vi "CR-字符检测处理函数as.vi"(0 "Image in":T6(plugin-control), 1 "字符识别参数":T5={"Parameters (OCR/OCV 1)"={"Threshold Data"={"Method"=enum."Local", "Looking for"=1, "Color Mode"=0, "Kernel Size"={"Width"=32, "Height"=32}, "Ranges"=[{"Min"=1, "Max"=255}]}, "Reject Border"=TRUE, "Number Of Erosions"=0, "Size & Spacing"={"Segment Algorithm"=0, "Min Bounding Rect Width"=1, "Max Bounding Rect Width"=65536, "Min Bounding Rect Height"=1, "Max Bounding Rect Height"=65536, "Min Character Size"=20, "Max Character Size"=65536, "Min Char Spacing"=1, "Max Horiz Element Spacing"=1, "Max Vert Element Spacing"=0, "Max Space Distance"=65536}, "Read Options"={"Read Strategy"=1, "Read Resolution"=2, "Scale Dependant"=FALSE, "Aspect Ratio"=400, "Acceptance Level"=700, "Substitution Character"="?", "MultiLine"=TRUE}, "Valid Characters"=[], "Use Text Pattern"=FALSE, "Orientation"=0, "# Lines Expected"=0, "Number of Blocks"=4}, "Rectangle"={"Left"=0, "Top"=0, "Right"=0, "Bottom"=0, "Rotation"=0.0}, "字符长度判定"=0.0, "Reference System"={"Origin"={"X"=1245.2058, "Y"=1038.7815}, "Angle (deg)"=0.021420227, "Axis Reference"=0}, "File Path (字符库)"=path "D:/Inspect System/Source Code/Template Program/字符模板.abc", "File Path (连接件模板)"=path "D:/Inspect System/Source Code/Template Program/字符检测定位模板.png", "Url"="http://10.6.1.31:8080/MesInnerpackLineIO.asmx", "accessKey"="a45b2d3334ffs_\na45b2d3334ffs_"} {"Reference System"."Axis Reference" items=["Direct", "Indirect"]; "Rectangle"."Rotation" min=-90.0 max=90.0 step=1.0 format="%.2f"; "Rectangle"."Left" scale=0.0..1024.0; "Rectangle"."Right" scale=0.0..1024.0; "Parameters (OCR/OCV 1)"."Threshold Data"."Looking for" items=["Light on Dark", "Dark on Light"]; "Parameters (OCR/OCV 1)"."Threshold Data"."Color Mode" items=["RGB", "HSL", "HSV", "HSI"]; "Parameters (OCR/OCV 1)"."Size & Spacing"."Segment Algorithm" items=["None", "Shortest Segment", "Legacy Auto Split"]; "Parameters (OCR/OCV 1)"."Read Options"."Read Strategy" items=["Aggressive", "Conservative"]; "Parameters (OCR/OCV 1)"."Read Options"."Read Resolution" items=["Low", "Medium", "High"]; "Parameters (OCR/OCV 1)"."Valid Characters"."Pre-defined characters" items=["Any Character", "User-defined Characters", "Alphabetic", "Alphanumeric", "Uppercase Letters", "Lowercase Letters", "Decimal Digits", "Hexadecimal Digits", "Pattern", "Force Space"]; "Parameters (OCR/OCV 1)"."Orientation" items=["Baseline inside", "Baseline outside"]}, 5 "error in (no error)":errorcluster caption="错误输入（无错误）", 7 "CCD1字符定位参数":T4={"Rectangle"={"Left"=9, "Top"=176, "Right"=891, "Bottom"=836, "Rotation"=0.0}, "Settings"={"Curve Parameters"={"Extraction Mode"=0, "Edge Threshold"=35, "Edge Filter Size"=1, "Min Length"=25, "Row Search Step Size"=15, "Col Search Step Size"=15, "Max Endpoint Gap"=10, "Closed"=FALSE, "Subpixel"=FALSE}, "Match Mode"={"Rotation"=TRUE, "Scale"=FALSE, "Occlusion"=TRUE, "Reserved 1"=FALSE, "Reserved 2"=FALSE, "Reserved 3"=FALSE}, "Range Settings"=[{"Match Constraints"=0, "Min"=-17.0, "Max"=17.0}], "Number of Matches"=1, "Minimum Match Score"=400.0, "SubPixel Accuracy"=FALSE, "Adv. Geometric Match Options 2"=[{"Setup Data Item"=21, "Item Value"=0.0}]}, "Template File Path"=path "D:/Inspect System/Source Code/SubVIs/字符检测VI/aaaa.png"} {"Settings"."Curve Parameters"."Extraction Mode" items=["Normal", "Uniform Regions"]; "Settings"."Curve Parameters"."Edge Filter Size" items=["Fine", "Normal", "Contour Tracing"]; "Settings"."Curve Parameters"."Max Endpoint Gap" min=0; "Settings"."Curve Parameters"."Col Search Step Size" min=1 max=255 step=1; "Settings"."Curve Parameters"."Row Search Step Size" min=1 max=255 step=1; "Settings"."Curve Parameters"."Min Length" min=0; "Settings"."Curve Parameters"."Edge Threshold" min=1 max=350 step=1; "Settings"."Range Settings"."Max" format="%.2f"; "Settings"."Range Settings"."Min" format="%.2f"; "Settings"."Range Settings"."Match Constraints" items=["Rotation Angle (degrees)", "Scale Factor (%)", "Occlusion (%)"]; "Settings"."Adv. Geometric Match Options 2"."Setup Data Item" items=["Curve Extraction Mode", "Curve Edge Threshold", "Curve Edge Filter Size", "Min Curve Length", "Curve Row Search Step Size", "Curve Col Search Step Size", "Curve Max Endpoint Gap", "Extract Closed Curves", "Enable Subpixel Curve Extraction", "Enable Correlation Score", "Enable Subpixel Accuracy", "Subpixel Iterations", "Subpixel Tolerance", "Initial Match List Length", "Enable Target Template Curve Score", "Min Match Separation Distance", "Min Match Separation Angle", "Min Match Separation Scale", "Max Match Overlap", "Enable Coarse Result", "Enable Calibration Support", "Enable Contrast Reversal", "Search Strategy", "Refinement Match Factor", "Subpixel Match Factor"]; "Rectangle"."Rotation" format="%.2f"; "Rectangle"."Left" scale=0.0..1024.0; "Rectangle"."Right" scale=0.0..1024.0}) -> (12 "模板匹配OK/NG":bool, 14 "Image out":T6(plugin-control), 16 "Data":string, 17 "字符方向判定结果":bool, 18 "结果":bool, 19 "error out":errorcluster caption="错误输出")   [LabVIEW 2017]
uses:
  <vilib>/vision/Pattern Matching.llb/IMAQ Curve Parameters.ctl
  <vilib>/vision/Pattern Matching.llb/IMAQ Match Range Setting.ctl
  <vilib>/vision/NI_Vision_Development_Module.lvlib
panel:
  in  "Bounding Box 3":cluster{"x":sgl, "y":sgl}[](array[cluster])
  out "Bounding Box 2":cluster{"x":sgl, "y":sgl}[](array[cluster])
  out "Bounding Box":cluster{"x":sgl, "y":sgl}[](array[cluster])
  # "D:\\Inspect System -2\\Source Code\\Template Program\\程序1\\字符模板.abc"
  # "Range"
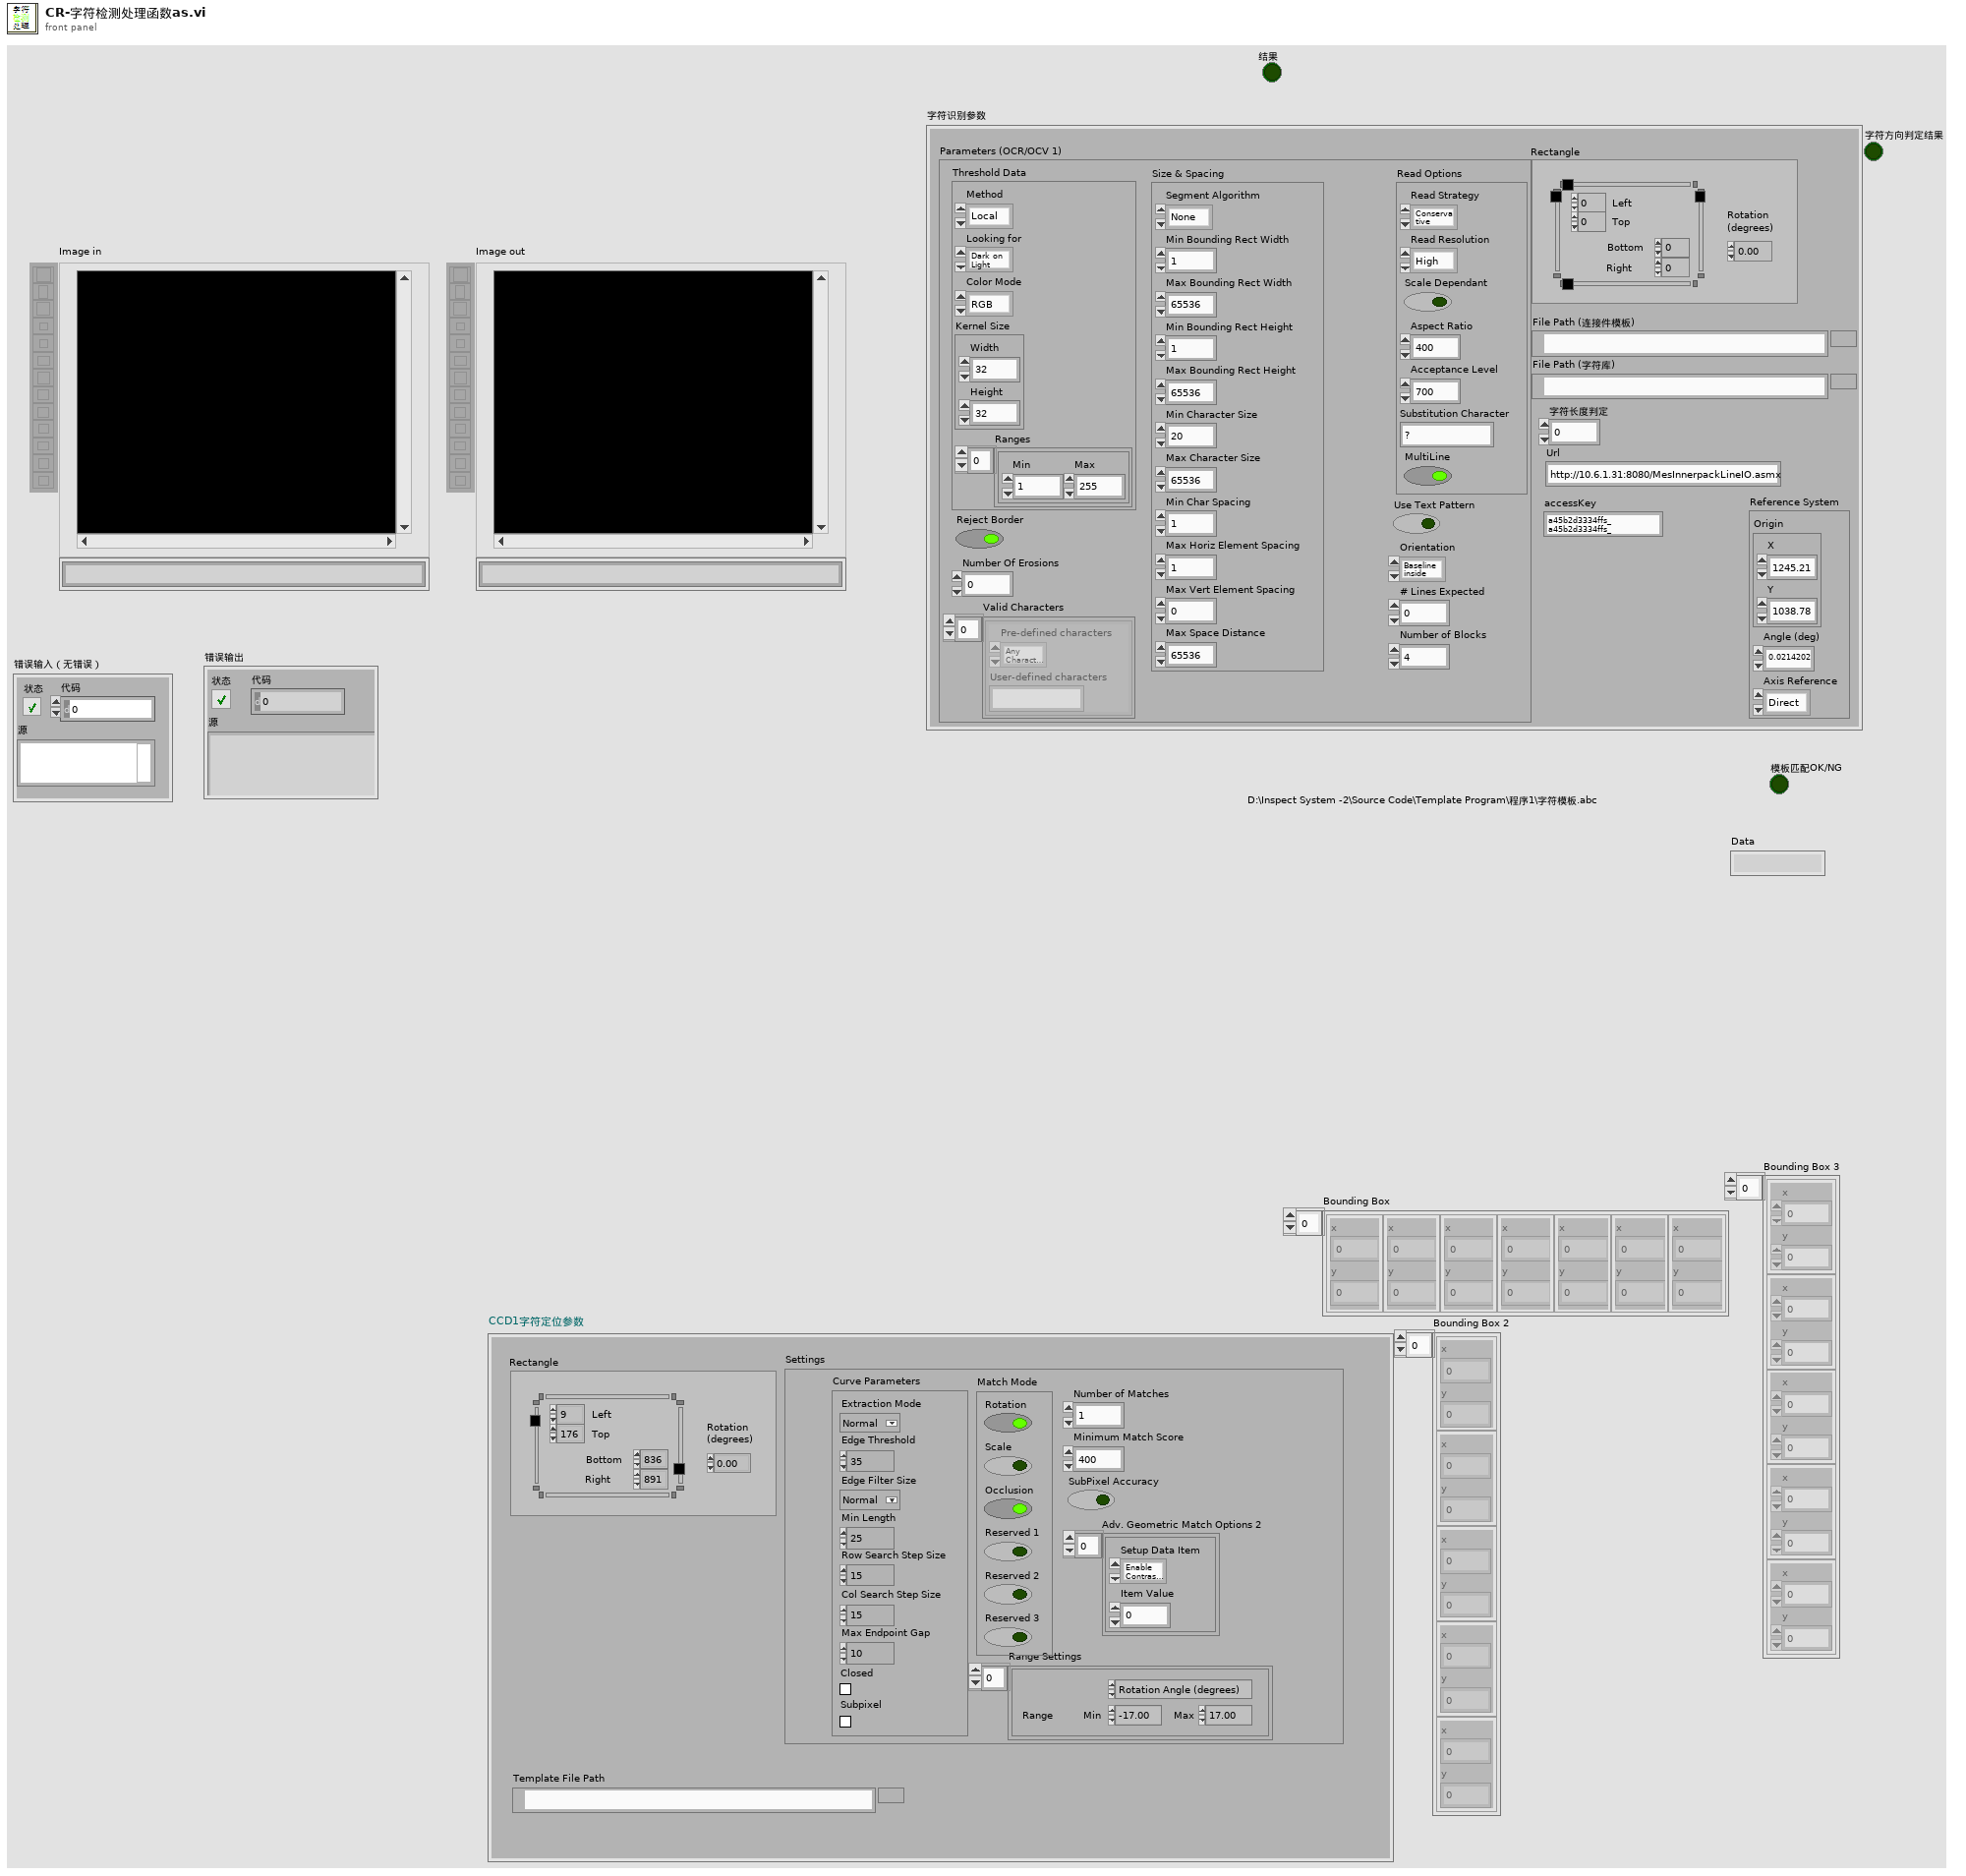
[diagram p1: front panel]
types:
  T1 = typedef "IMAQ Rectangle" = cluster{"Left":i32, "Top":i32, "Right":i32, "Bottom":i32, "Rotation":dbl}
  T2 = typedef "IMAQ Curve Parameters.ctl" = cluster{"Extraction Mode":u32, "Edge Threshold":i32, "Edge Filter Size":u32, "Min Length":i32, "Row Search Step Size":i32, "Col Search Step Size":i32, "Max Endpoint Gap":i32, "Closed":bool, "Subpixel":bool}
  T3 = typedef "IMAQ Match Range Setting.ctl" = cluster{"Match Constraints":u32, "Min":dbl, "Max":dbl}
  T4 = cluster{"Rectangle":T1, "Settings":cluster{"Curve Parameters":T2, "Match Mode":cluster{"Rotation":bool, "Scale":bool, "Occlusion":bool, "Reserved 1":bool, "Reserved 2":bool, "Reserved 3":bool}, "Range Settings":T3[], "Number of Matches":i32, "Minimum Match Score":sgl, "SubPixel Accuracy":bool, "Adv. Geometric Match Options 2":cluster{"Setup Data Item":u16, "Item Value":dbl}[]}, "Template File Path":path}
  T5 = cluster{"Parameters (OCR/OCV 1)":cluster{"Threshold Data":cluster{"Method":enum16{"Fixed Range", "Uniform", "Linear", "Non Linear", "Local", "Color"}, "Looking for":u32, "Color Mode":u32, "Kernel Size":cluster{"Width":i32, "Height":i32}, "Ranges":cluster{"Min":i32, "Max":i32}[]}, "Reject Border":bool, "Number Of Erosions":i32, "Size & Spacing":cluster{"Segment Algorithm":u16, "Min Bounding Rect Width":i32, "Max Bounding Rect Width":i32, "Min Bounding Rect Height":i32, "Max Bounding Rect Height":i32, "Min Character Size":i32, "Max Character Size":i32, "Min Char Spacing":i32, "Max Horiz Element Spacing":i32, "Max Vert Element Spacing":i32, "Max Space Distance":i32}, "Read Options":cluster{"Read Strategy":i32, "Read Resolution":i32, "Scale Dependant":bool, "Aspect Ratio":i32, "Acceptance Level":i32, "Substitution Character":string, "MultiLine":bool}, "Valid Characters":cluster{"Pre-defined characters":i32, "User-defined characters":string}[], "Use Text Pattern":bool, "Orientation":u32, "# Lines Expected":u32, "Number of Blocks":i32}, "Rectangle":T1, "字符长度判定":dbl, "Reference System":cluster{"Origin":cluster{"X":sgl, "Y":sgl}, "Angle (deg)":sgl, "Axis Reference":u32}, "File Path (字符库)":path, "File Path (连接件模板)":path, "Url":string, "accessKey":string}
  T6 = typedef "IMAQ Image.ctl" = refnum<image>
  T7 = cluster{"Rotation Mode":enum32{"Unlimited", "0 Degrees", "90 Degrees", "180 Degrees", "270 Degrees"}, "Skip Location?":bool, "Edge Threshold":u32, "Demodulation Mode":i32, "Cell Sample Size":i32, "Cell Filter Mode":i32, "Skew Degrees Allowed":u32}
  T8 = cluster{"Left":i32, "Top":i32, "Right":i32, "Bottom":i32}
  T9 = cluster{"Global Rectangle":i32[], "Contours":cluster{"ID":enum32{"External", "Internal"}, "Type":u32, "Coordinates":i32[]}[]}
  T10 = cluster{"Desired Font (Application)":enum16{"User-specified Font", "Application Font", "System Font", "Dialog Font"}, "[User-specified Font]":cluster{"Font Name":string, "Size":i16, "Strikeout?":bool, "Italic?":bool, "Underline?":bool, "Outline?":bool, "Shadow?":bool, "Bold?":bool, "Rotation Angle":dbl}, "Horizontal Alignment":i16, "Vertical Alignment":i16}
  T11 = typedef "ROI Descriptor" = cluster{"Global Rectangle":i32[], "Contours":cluster{"ID":enum32{"External", "Internal"}, "Type":u32, "Coordinates":i32[]}[]}
  T12 = typedef "IMAQ GM Match Report.ctl" = cluster{"Position":cluster{"x":sgl, "y":sgl}, "Angle":sgl, "Scale":sgl, "Score":sgl, "Bounding Box":cluster{"x":sgl, "y":sgl}[], "Contrast Reversed":bool, "Occlusion %":sgl, "Template Target Curve Score":sgl, "Target Template Curve Score":sgl, "Correlation Score":sgl}
  T13 = cluster{"Reference System":cluster{"Origin":cluster{"X":sgl, "Y":sgl}, "Angle (deg)":sgl, "Axis Reference":u32}, "Measurement System":cluster{"Origin":cluster{"X":sgl, "Y":sgl}, "Angle (deg)":sgl, "Axis Reference":u32}}
  T14 = cluster{"Position":cluster{"x":sgl, "y":sgl}, "Angle":sgl, "Scale":sgl, "Score":sgl, "Bounding Box":cluster{"x":sgl, "y":sgl}[]}[]
  T15 = cluster{"Position":cluster{"x":sgl, "y":sgl}, "Angle":sgl, "Scale":sgl, "Score":sgl, "Bounding Box":cluster{"x":sgl, "y":sgl}[]}
  T16 = cluster{"Origin":cluster{"X":sgl, "Y":sgl}, "Angle (deg)":sgl, "Axis Reference":u32}
  T17 = typedef "QR Code Report.ctl" = cluster{"Found?":bool, "Data":string, "Bounding Box":cluster{"x":sgl, "y":sgl}[], "Errors Corrected":u32, "Dimensions (Rows/Cols)":u32, "Version":u32, "QR Model":T18, "Stream Mode":T19, "Barcode Polarity":T20, "Mirrored?":bool, "Append Stream Position":u32, "Size of Append Stream":u32, "First EAN-128 ID":i32, "First Alternate Language ID":i32, "Append Stream ID":u32, "Minimum Edge Strength":u32, "Demodulation Mode":T21, "Cell Sample Size":T22, "Cell Filter Mode":T23}
  T18 = typedef "QR Code Model Type.ctl" = i32
  T19 = typedef "QR Code Stream Mode Type.ctl" = i32
  T20 = typedef "Data Matrix Polarity.ctl" = i32
  T21 = typedef "Demodulation Mode.ctl" = i32
  T22 = typedef "Cell Sample Size.ctl" = i32
  T23 = typedef "Cell Filter Mode.ctl" = i32
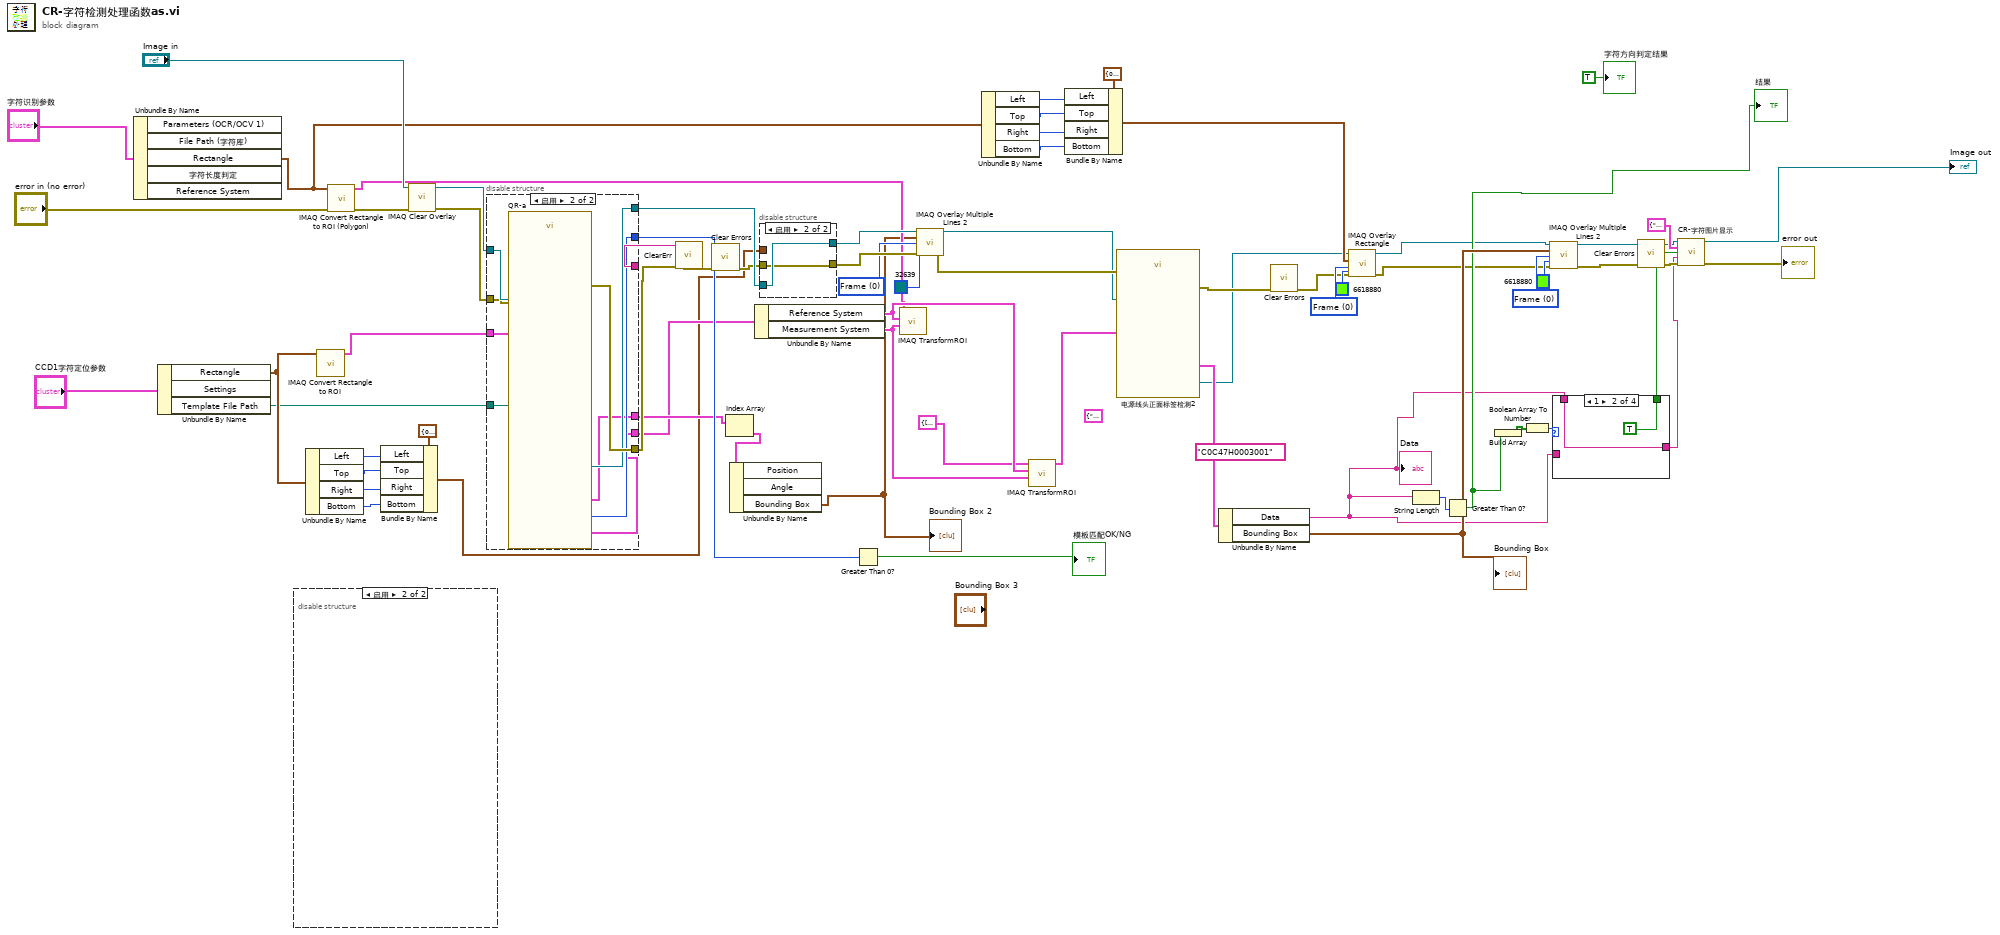
[diagram p0: block diagram]
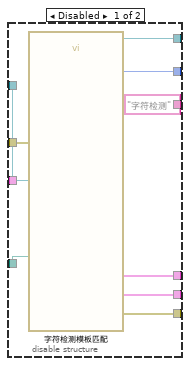
[diagram p2: hidden frame]
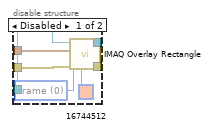
[diagram p3: hidden frame]
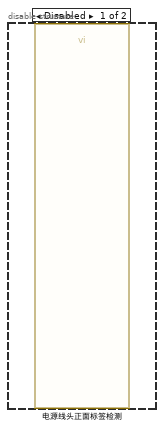
[diagram p4: hidden frame]
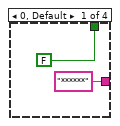
[diagram p5: hidden frame]
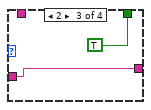
[diagram p6: hidden frame]
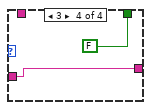
[diagram p7: hidden frame]
diagram:
  (unwired) T7 {"Rotation Mode"=enum."Unlimited", "Skip Location?"=FALSE, "Edge Threshold"=11, "Demodulation Mode"=1, "Cell Sample Size"=3, "Cell Filter Mode"=2, "Skew Degrees Allowed"=5} ("QR Search Options (2D Barcode Reader 1)")
  w20 = u32 0 items=["Frame", "Fill"] ("Drawing Mode (Frame)")
  w22 = u32 0 items=["Frame", "Fill"] ("Drawing Mode (Frame)")
  (unwired) "C0C47H0003001" ("Data")
  w57 = u32 0 items=["Frame", "Fill"] ("Drawing Mode (Frame)")
  n1 = Unbundle By Name("字符识别参数") -> ("Rectangle"=w5:T1)  [unwired: 4 out]
  n2 = Unbundle By Name("CCD1字符定位参数") -> ("Rectangle"=w41:T1, "Template File Path"=w33:path)  [unwired: 1 out]
  n3 = disable-structure shown="启用" {
    frame Disabled {
      n4 = call "电源线头正面标签检测"() -> ()  [unwired: 21 in, 7 out]
    }
    frame Enabled {
    }
  }
  n5 = Unbundle By Name(w41) -> ("Left"=w40:i32, "Top"=w39:i32, "Right"=w38:i32, "Bottom"=w37:i32)
  n6 = call "IMAQ Convert Rectangle to ROI"("Rectangle"=w41) -> ("ROI Descriptor"=w15:T11)  [unwired: 8 in, 1 out]
  n7 = call "IMAQ Convert Rectangle to ROI (Polygon)"("error in (no error)"="error in (no error)", "Rectangle"=w5) -> ("error out"=w45:errorcluster, "ROI Descriptor"=w13:T11)  [unwired: 6 in, 1 out]
  n8 = Bundle By Name(cluster=T8 {"Left"=0, "Top"=0, "Right"=0, "Bottom"=0} ("Rectangle"), "Left"=w40, "Top"=w39, "Right"=w38, "Bottom"=w37) -> (w11:T8)
  n9 = call "IMAQ Clear Overlay"("error in (no error)"=w45, "Image"="Image in") -> ("error out"=w34:errorcluster, "Image Out"=w28:T6)  [unwired: 8 in]
  n10 = disable-structure shown="启用" {
    disable-tunnel: [w79 w83] -> w63
    disable-tunnel: ["字符检测" ("运行位置") _] -> w36
    disable-tunnel: w34 -> [w77 w86]
    disable-tunnel: w33 -> [w76 w88]
    disable-tunnel: [w75 w85] -> w32
    disable-tunnel: [w74 w81] -> w31
    disable-tunnel: [w73 w82] -> w30
    disable-tunnel: [w72 w84] -> w29
    disable-tunnel: w28 -> [w71 w87]
    disable-tunnel: w15 -> [_ w80]
    frame Disabled {
      n11 = call "字符检测模板匹配.vi"("Image In"=w71, "Template File Path (Geometric Matching 1)"=w76, "error in"=w77) -> ("Image Out"=w72:T6, "Calibrated Matches (Geometric Matching 1)"=w74:T12[], "Number of Matches (Geometric Matching 1)"=w79:i32, "Coordinate System Out (Set Coordinate System 1)"=w73:T13, "error out"=w75:errorcluster)  [unwired: 19 in, 1 out]
    }
    frame Enabled {
      n12 = call "QR-a.vi"("Image In"=w87, "Template File Path (Pattern Matching 1)"=w88, "error in"=w86, "ROI Descriptor (2D Barcode Reader 1)"=w80) -> ("Image Out"=w84:T6, "Calibrated Matches (Pattern Matching 1)"=w81:T14, "Number of Matches (Pattern Matching 1)"=w83:i32, "Coordinate System Out (Set Coordinate System 1)"=w82:T13, "error out"=w85:errorcluster)  [unwired: 16 in, 3 out]
    }
  }
  n13 = call "ClearErr.vi"("error in (no error)"=w32, "运行位置"=w36) -> ("error out"=w35:errorcluster)  [unwired: 9 in]
  n14 = call <vilib>:"Clear Errors.vi"("error in (no error)"=w35) -> ("error out"=w24:errorcluster)  [unwired: 5 in, 1 out]
  n15 = Index Array(array=w31) -> (element=w44:T15)  [unwired: 1 in]
  n16 = Unbundle By Name(w44) -> ("Bounding Box"=w1:cluster{"x":sgl, "y":sgl}[])  [unwired: 2 out]
  "Bounding Box 2" <- w1
  n17 = Unbundle By Name(w30) -> ("Reference System"=w26:T16, "Measurement System"=w27:T16)
  n18 = disable-structure shown="启用" {
    disable-tunnel: w11 -> [w95 _]
    disable-tunnel: w29 -> [w94 w97]
    disable-tunnel: [w93 w97] -> w25
    disable-tunnel: w24 -> [w92 w96]
    disable-tunnel: [w89 w96] -> w23
    frame Disabled {
      w91 = u32 0 items=["Frame", "Fill", "Highlight"] ("Drawing Mode (Frame)")
      n19 = call "IMAQ Overlay Rectangle"("Color"=u32 16744512, "error in (no error)"=w92, "Drawing Mode (Frame)"=w91, "Rectangle"=w95, "Image"=w94) -> ("error out"=w89:errorcluster, "Image Out"=w93:T6)  [unwired: 5 in]
    }
    frame Enabled {
    }
  }
  n20 = Greater Than 0?(x=w63) -> (x > 0?=→"模板匹配OK/NG":bool)
  n21 = call "IMAQ TransformROI"("New Reference"=w27, "Base Reference"=w26, "ROI Descriptor"=w13) -> ()  [unwired: 7 in, 2 out]
  n22 = call "IMAQ Overlay Multiple Lines 2"("Image"=w25, "Line End Points"=w1, "Drawing Mode (Frame)"=w22, "Color"=u32 32639, "error in (no error)"=w23) -> ("Image Out"=w62:T6, "error out"=w66:errorcluster)  [unwired: 9 in]
  n23 = Unbundle By Name(w5) -> ("Left"=w9:i32, "Top"=w8:i32, "Right"=w7:i32, "Bottom"=w6:i32)
  n24 = call "IMAQ TransformROI"("New Reference"=w27, "Base Reference"=w26, "ROI Descriptor"=T9 {"Global Rectangle"=[579, 508, 906, 745], "Contours"=[{"ID"=enum."External", "Type"=3, "Coordinates"=[579, 508, 906, 745]}]} ("ROI Descriptor (2D Barcode Reader 1)")) -> ("ROI Descriptor out"=w14:T11)  [unwired: 7 in, 1 out]
  n25 = Bundle By Name(cluster=T8 {"Left"=0, "Top"=0, "Right"=0, "Bottom"=0} ("Rectangle"), "Left"=w9, "Top"=w8, "Right"=w7, "Bottom"=w6) -> (w4:T8)
  n26 = call "电源线头正面标签检测2"("Image In"=w62, "error in"=w66, "ROI Descriptor (2D Barcode Reader 1)"=w14) -> ("Image Out"=w3:T6, "QR Barcode Report (2D Barcode Reader 1)"=w61:T17, "error out"=w50:errorcluster)  [unwired: 22 in]
  n27 = Unbundle By Name(w61) -> ("Data"=w2:string, "Bounding Box"=w56:cluster{"x":sgl, "y":sgl}[])
  "Data" <- w2
  "Bounding Box" <- w56
  n28 = call <vilib>:"Clear Errors.vi"("error in (no error)"=w50) -> ("error out"=w18:errorcluster)  [unwired: 5 in, 1 out]
  n29 = call "IMAQ Overlay Rectangle"("Color"=u32 6618880, "error in (no error)"=w18, "Drawing Mode (Frame)"=w20, "Rectangle"=w4, "Image"=w3) -> ("error out"=w17:errorcluster, "Image Out"=w16:T6)  [unwired: 5 in]
  n30 = String Length(string=w2) -> (length=w55:i32)
  n31 = Greater Than 0?(x=w55) -> (x > 0?=w48:bool)
  "结果" <- w48
  n32 = Build Array(w48) -> (w52:bool[])
  n33 = Boolean Array To Number(Boolean array=w52) -> (number=w53:u32)
  n34 = call "IMAQ Overlay Multiple Lines 2"("Image"=w16, "Line End Points"=w56, "Drawing Mode (Frame)"=w57, "Color"=u32 6618880, "error in (no error)"=w17) -> ("Image Out"=w58:T6, "error out"=w59:errorcluster)  [unwired: 9 in]
  n35 = case shown="1" w53 {
    tunnel: ["******" ("Data") w101 w103 w105] -> w54
    tunnel: w2 -> [_ w101 _ _]
    tunnel: w2 -> [_ _ w103 w105]
    tunnel: [FALSE TRUE TRUE FALSE] -> w51
    frame 0, Default {
    }
    frame 1 {
    }
    frame 2 {
    }
    frame 3 {
    }
  }
  n36 = call <vilib>:"Clear Errors.vi"("error in (no error)"=w59) -> ("error out"=w68:errorcluster)  [unwired: 5 in, 1 out]
  n37 = call "CR-字符图片显示.vi"("Image in"=w58, "Font, Size & Style"=T10 {"Desired Font (Application)"=enum."User-specified Font", "[User-specified Font]"={"Font Name"="", "Size"=50, "Strikeout?"=FALSE, "Italic?"=FALSE, "Underline?"=FALSE, "Outline?"=FALSE, "Shadow?"=FALSE, "Bold?"=TRUE, "Rotation Angle"=0.0}, "Horizontal Alignment"=0, "Vertical Alignment"=0}, "是否检测到字符串"=w51, "String (OCR/OCV 1)"=w54, "error in (no error)"=w68) -> ("Image out"=→"Image out":T6, "error out"=→"error out":errorcluster)  [unwired: 9 in]
  "字符方向判定结果" <- TRUE ("字符方向判定结果")
